vi "ColourPalleteExample.vi"() -> ()   [LabVIEW 2023]
uses:
  repositories/egen3/me/multisim/labview_gui/source/Typedefs/ME_ControlStation/CommunicationPanel.ctl
  repositories/egen3/me/appfrdev/labview_gui/source/Support_Libs/Application/FP_Config.ctl
  repositories/egen3/me/multisim/labview_gui/source/Typedefs/ME_ControlStation/ControlStationConfiguration.ctl
panel:
  in  "ECR":bool=TRUE
  out "Numeric":dbl
  in  "Tab Control 3":enum32{"Page 1", "Page 2"}(tab)
  in  "Tab Control 4":enum32{"Page 1", "Page 2"}(tab)
  in  "Tab Control 5":enum32{"Page 1", "Page 2"}(tab)
  in  "Tab Control 2":enum32{"Page 1", "Page 2"}(tab)
  out "Tab Control":enum32{"VISIBLE", "INVISIBLE"}(tab)
  out "Configuration Options":T1
  in  "pytest_speedset":dbl
  in  "pytest_stop_labview":dbl
  in  "polling_speed":i32=100
  in  "Stop":bool caption="_Stop"
  in  "error in (no error)":errorcluster
  out "error out":errorcluster
  in  "FP Window Config":T2={"Width"=1500, "Height"=930, "Unlocked?"=FALSE}
  out "Testwall status tab control":enum32{"Enabled", "Disabled"}(tab)
  in  "mcs_controller_status":bool caption="Caption"
  in  "mcs_io_interface":bool caption="Caption"
  in  "mcs_testwall_status":bool caption="Caption"
  in  "Grow Button":bool
  in  "Shrink Button":bool
  in  "Emergency Stop LOP":bool caption="Caption"
  in  "Emergency Stop Bridge":bool caption="Caption"
  out "I&C Panel":T3(tab)
  out "Bridge_StartAirPressureLow":bool caption="Start Air Pressure Low"
  out "Bridge_StartAirPressure":dbl caption="Start Air Pressure [Bar]" format="%#.2f"
  out "Bridge_StartFailed":bool caption="Start failed"
  out "Bridge_RepeatedStart":bool caption="Repeated Start"
  out "Bridge_Delayed Start":bool caption="Delayed Start"
  out "Bridge_PreparingStart":bool caption="Preparing Start"
  out "Bridge_EngineNotReady":bool caption="Engine Not Ready"
  out "Bridge_FixedLoadLim":dbl caption="Fixed Load Limit [%]" format="%#.2f"
  out "Bridge_LimitationIncreased":bool caption="Limitation Increased"
  in  "Bridge_Increase Limits":bool caption="Caption"
  out "Bridge_Load Limitation":bool caption="Load Limitation"
  in  "Bridge_PrepareTierIII":bool caption="Caption"
  out "Bridge_DFStatus":dbl caption="Dual Fuel Status" format="%#.2f"
  out "Bridge_TierIIISystemStatus":dbl caption="Tier III System Status" format="%#.2f"
  out "Bridge_SelectedEngineMode":dbl caption="Selected Engine Mode" format="%#.2f"
  out "Bridge_Second Fuel Mode":bool caption="Second Fuel Mode"
  out "Bridge_ShutDown Prewarning":bool caption="ShutDown Prewarning"
  out "Bridge_ShutDown Cancelled":bool caption="ShutDown Cancelled"
  in  "Bridge_Cancel ShutDown":bool caption="Caption"
  out "Bridge_ShutDown Active":bool caption="ShutDown Active"
  in  "Bridge_Cancel SlowDown":bool caption="Caption"
  in  "Bridge_Reset SlowDown":bool caption="Caption"
  out "Bridge_SlowDown Prewarning":bool caption="SlowDown Prewarning"
  out "Bridge_SlowDown Active":bool caption="SlowDown Active"
  out "Bridge_SlowDown Cancelled":bool caption="SlowDown Cancelled"
  in  "ECR_Increase Limits":bool caption="Caption"
  out "ECR_Load Limitation":bool caption="Load Limitation"
  in  "ECR_Cancel ShutDown":bool caption="Caption"
  out "ECR_ShutDown Active":bool caption="ShutDown Active"
  out "ECR_ShutDown Cancelled":bool caption="ShutDown Cancelled"
  out "ECR_ShutDown Prewarning":bool caption="ShutDown Prewarning"
  in  "ECR_Cancel SlowDown":bool caption="Caption"
  in  "ECR_Reset SlowDown":bool caption="Caption"
  out "ECR_SlowDown Cancelled":bool caption="SlowDown Cancelled"
  out "ECR_SlowDown Prewarning":bool caption="SlowDown Prewarning"
  out "ECR_SlowDown Active":bool caption="SlowDown Active"
  out "LOP_HydraulicPressure":dbl caption="Hydraulic Pressure [Bar]" format="%#.2f"
  out "LOP_AuxBlowersWarning":bool caption="Aux. Blowers Warning"
  out "LOP_AuxBlowersRunning":bool caption="Aux. Blowers Running"
  out "LOP_TurningGearDisengaged":bool caption="Turning Gear Disengaged"
  out "LOP_MainStartValveInPos":bool caption="Main Start Valve In Position"
  out "LOP_StartAirDistInService":bool caption="Start Air Dist. In Service"
  out "LOP_Startfailed":bool caption="Start failed"
  out "LOP_StartAirPressure":dbl caption="Start Air Pressure [Bar]" format="%#.2f"
  out "LOP_StartBlock":bool caption="Start blocked"
  out "LOP_EngineNotReady":bool caption="Engine Not Ready"
  out "LOP_LimitationIncreased":bool caption="Limitation Increased"
  out "LOP_Load Limitation":bool caption="Load Limitation"
  in  "LOP_Increase Limits":bool caption="Caption"
  in  "SF Shutdown LOP":bool caption="Caption"
  out "LOP_Second Fuel Mode":bool caption="Second Fuel Mode"
  out "LOP_ShutDown Prewarning":bool caption="ShutDown Prewarning"
  out "LOP_ShutDown Cancelled":bool caption="ShutDown Cancelled"
  in  "LOP_Cancel ShutDown":bool caption="Caption"
  out "LOP_ShutDown Active":bool caption="ShutDown Active"
  in  "LOP_Cancel SlowDown":bool caption="Caption"
  in  "LOP_Reset SlowDown":bool caption="Caption"
  out "LOP_SlowDown Prewarning":bool caption="SlowDown Prewarning"
  out "LOP_SlowDown Active":bool caption="SlowDown Active"
  out "LOP_SlowDown Cancelled":bool caption="SlowDown Cancelled"
  in  "mcs_CtrlStation I&C":T4 items=["ENGINE CONDITION & START", "LIMITATIONS", "ENGINE MODE", "SAFETY SYSTEM /SHUTDOWN", "SLOWDOWN", "WRONG WAY ALARM"]
  in  "Force_Take_LOP":bool caption="Caption"
  out "Engine Blocked":bool
  out "Engine Ready":bool
  out "FWE":bool caption="Status ON/OFF"
  out "Standby":bool caption="Status ON/OFF"
  out "AtSea":bool caption="Status ON/OFF"
  in  "Emergency Stop ECR":bool caption="Caption"
  in  "SF Shutdown":bool caption="Caption"
  in  "Force_Take_ECR":bool caption="Caption"
  out "LOP_In_Command":bool caption="Status ON/OFF"
  out "ECR_In_Command":bool=TRUE caption="Status ON/OFF"
  out "Bridge_In_Command":bool caption="Status ON/OFF"
  out "LOP Forced":bool
  out "ECR Forced":bool
  out "ECR_Sep_In_Command":bool caption="Status ON/OFF"
  in  "LOP_Request":bool caption="Caption"
  in  "ECR_Request":bool caption="Caption"
  in  "Bridge_Request":bool caption="Caption"
  in  "ECR_Sep_Request":bool caption="Caption"
  in  "AtSea_Request":bool caption="Caption"
  in  "Standby_Request":bool caption="Caption"
  in  "FWE_Request":bool caption="Caption"
  in  "Seperator SP":dbl(slide) caption="Seperator Setpoint" min=-250.0 max=250.0 step=1.0 scale=0.0..100.0
  in  "mcs_CtrlStation":enum32{"LOP", "Bridge"}(radio)=enum."Bridge"
  in  "Start Engine":bool caption="Caption"
  in  "Speed Up":bool caption="Caption"
  in  "Speed Down":bool caption="Caption"
  in  "Stop Engine":bool caption="Caption"
  out "Pitch Indicator":enum32{"Enabled", "Disabled"}(tab)
  out "Pitch 2":dbl(knob) caption="PITCH" scale=-100.0..100.0
  out "Scavenge Air":dbl(slide) scale=0.0..4.0
  out "Start Air":dbl(slide) scale=0.0..30.0
  out "Inlet Oil":dbl(slide) scale=0.0..10.0
  out "Hydraulic Oil":dbl(slide) scale=150.0..325.0
  out "Governor Index":dbl(knob) caption="GOV. INDEX" scale=0.0..120.0
  out "Engine Speed":dbl(knob) caption="ENGINE SPEED" scale=-250.0..250.0
  out "ShrunkenArea":bool
  # "CONTROL STATION"
  # "LOP"
  # "RPM"
  # "%"
  # "Control Station"
  # "Operational State"
  # "ECR"
  # "Emergency Stop"
  # "Only used un Pytest"
  # "Press status buttons for more info..."
  # "TESTWALL STATUS"
  # "%"
  # "INDICATION & COMMUNICATION PANEL"
  # "PROPULSION CONTROL"
  # "KEY VALUES"
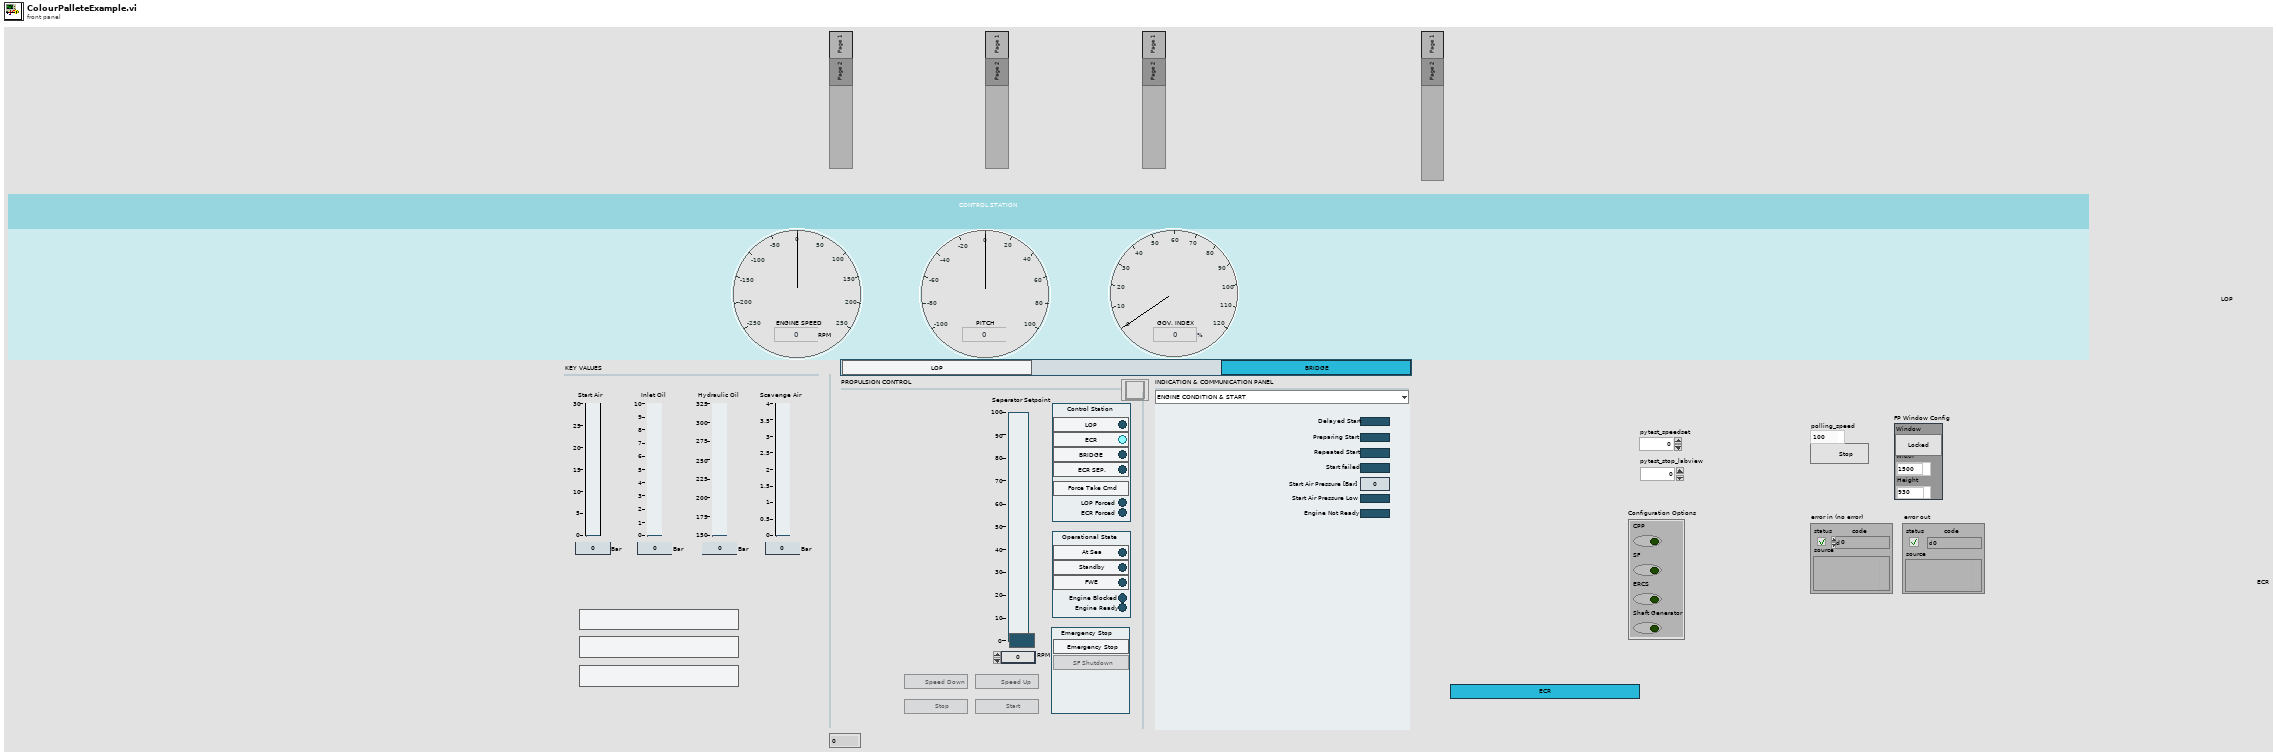
[diagram p1: front panel]
types:
  T1 = typedef "ControlStationConfiguration.ctl" = cluster{"CPP":bool, "SF":bool, "ERCS":bool, "Shaft Generator":bool}
  T2 = typedef "Application.lvlib/FP_Config.ctl" = cluster{"Width":i16, "Height":i16, "Unlocked?":bool}
  T3 = enum32{"Bridge - ENGINE CONDITION & START", "Bridge - LIMITATIONS", "Bridge - ENGINE MODE", "Bridge - SAFETY SYSTEM / SHUTDOWN", "Bridge - SLOWDOWN", "Bridge - WRONG WAY ALARM", "Bridge - CPP", "Bridge - EEXI", "Bridge - SHAFT GENERATOR", "ECR - ENGINE CONDITION & START", "ECR - LIMITATIONS", "ECR - ENGINE MODE", "ECR - SAFETY SYSTEM / SHUTDOWN", "ECR - SLOWDOWN", "ECR - WRONG WAY ALARM", "ECR - CPP", "ECR - EEXI", "ECR - SHAFT GENERATOR", "LOP - ENGINE CONDITION & START", "LOP - LIMITATIONS", "LOP - ENGINE MODE", "LOP - SAFETY SYSTEM / SHUTDOWN", "LOP - SLOWDOWN", "LOP - WRONG WAY ALARM", "LOP - CPP", "LOP - EEXI", "LOP - SHAFT GENERATOR"}
  T4 = typedef "CommunicationPanel.ctl" = u16
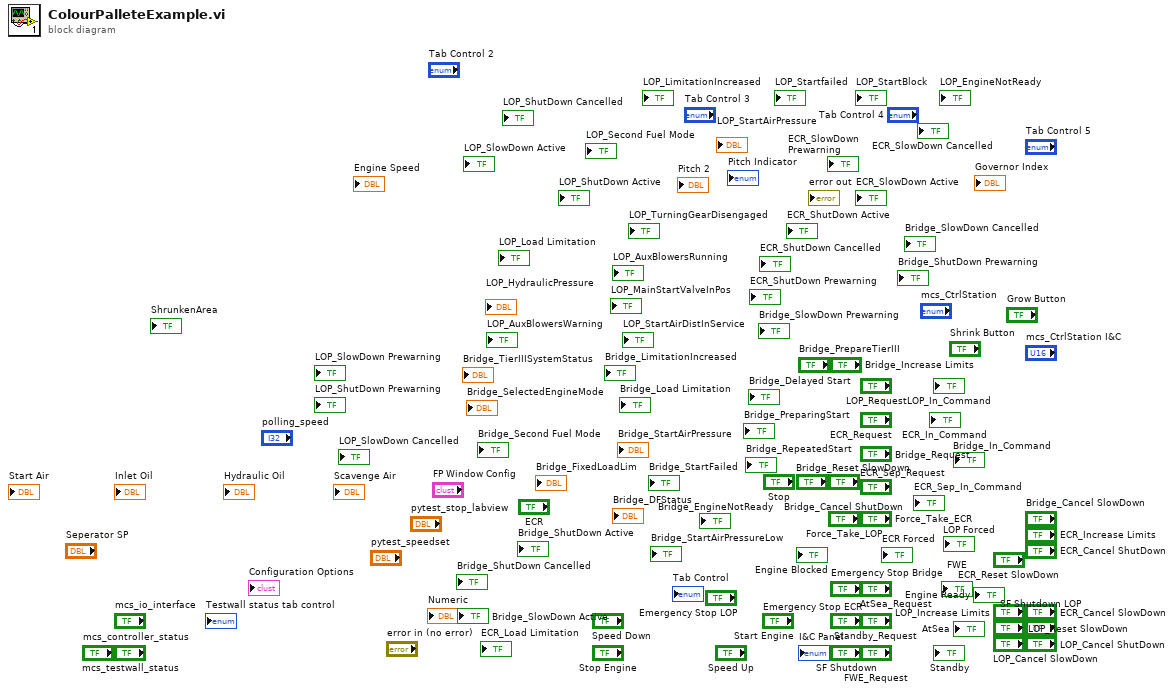
[diagram p0: block diagram]
diagram:
